vi "FTW-WebServer-Worker.vi"(1 "Endpoint":refnum<class "FTW-Endpoint.lvclass">, 2 "Message Handler":refnum<user-event>) -> ()   [LabVIEW 2015, in "FTW-WebServer.lvclass"]
uses:
  FTW-WebServer.lvclass
  Endpoint/FTW-Endpoint.lvclass
  Message/HttpRequest/FTW-Message-HttpRequest.lvclass
panel:
  out "Messages Handled":u32
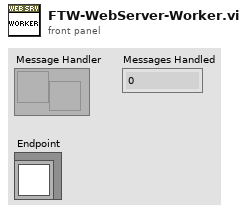
[diagram p1: front panel]
types:
  T1 = typedef "FTW-MessagePayload.ctl" = cluster{"Header":string, "Body":string, "FTW: Sender Identity":string, "FTW: Reply Address":string, "FTW: Reply Error":errorcluster}
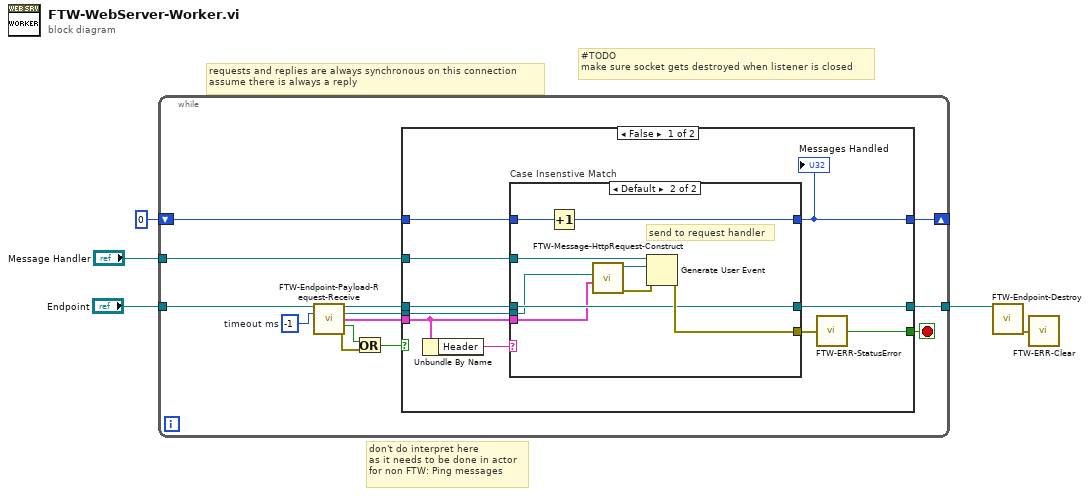
[diagram p0: block diagram]
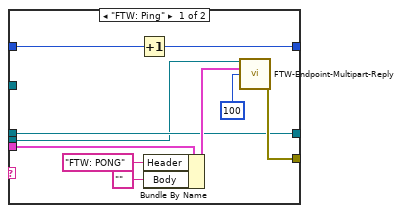
[diagram p2: hidden frame]
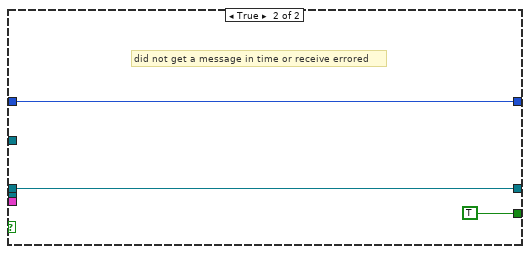
[diagram p3: hidden frame]
diagram:
  # "don't do interpret here\nas it needs to be done in actor\nfor non FTW: Ping messages"
  # "#TODO\nmake sure socket gets destroyed when listener is closed"
  # "requests and replies are always synchronous on this connection\nassume there is always a reply"
  n1 = while {
    tunnel: "Message Handler" -> [w18]
    shift-right: [w11] -> _
    shift-left: u32 0 -> [w12]
    tunnel: "Endpoint" -> [w17]
    tunnel: [w8] -> w3
    stop <- w13 stop-if-true
    w16 = -1  # timeout ms
    n2 = call-dynamic "FTW-Endpoint-Payload-Request-Receive.vi"("FTW Endpoint"=w17, "Timeout"=w16) -> ("FTW Endpoint out"=w10:refnum<class "FTW-Endpoint.lvclass">, "Reply Endpoint"=w14:refnum<class "FTW-Endpoint.lvclass">, "Payload"=w6:T1, "Timed out?"=w7:bool, "error out"=w15:errorcluster)  [unwired: 9 in]
    n3 = Or(x=w7, y=w15) -> (x .or. y?=w9:bool)
    n4 = case shown="False" w9 {
      tunnel: w18 -> [w28 _]
      tunnel: w14 -> [w21 _]
      tunnel: [w24 TRUE] -> w13
      tunnel: w10 -> [w25 w48]
      tunnel: w12 -> [w27 w50]
      tunnel: [w22 w50] -> w11
      tunnel: [w23 w48] -> w8
      tunnel: w6 -> [w20 _]
      frame False {
        n5 = Unbundle By Name(w20) -> ("Header"=w19:string)
        n6 = case "Case Insenstive Match" shown="Default" w19 {
          tunnel: w28 -> [_ w47]
          tunnel: w27 -> [w38 w46]
          tunnel: [w35 w45] -> w22
          tunnel: [w37 w42] -> w26
          tunnel: w25 -> [w31 w41]
          tunnel: w21 -> [w30 w40]
          tunnel: [w31 w41] -> w23
          tunnel: w20 -> [w32 w39]
          frame "FTW: Ping" {
            n7 = Increment(x=w38) -> (x+1=w35:u32)
            n8 = Bundle By Name(cluster=w32, "Header"="FTW: PONG" ("Part"), "Body"="" ("empty string")) -> (w34:T1)
            n9 = call-dynamic "FTW-Endpoint-Multipart-Reply.vi"("FTW Endpoint"=w30, "Message"=w34, "Timeout"=100) -> ("error out"=w37:errorcluster)  [unwired: 10 in, 2 out]
          }
          frame Default {
            # "send to request handler"
            n10 = Increment(x=w46) -> (x+1=w45:u32)
            n11 = call "FTW-Message-HttpRequest-Construct.vi"("Message"=w39, "Frontend Endpoint"=w40) -> ("error out"=w44:errorcluster, "FTW Incoming Request"=w43:refnum<class "FTW-Message-HttpRequest.lvclass">)  [unwired: 8 in]
            n12 = Generate User Event(user event=w47, event data cluster=w43, error in=w44) -> (error out=w42:errorcluster)  [unwired: 1 in, 1 out]
          }
        }
        "Messages Handled" <- w22
        n13 = call "FTW-ERR-StatusError.vi"("error to check"=w26) -> ("Error?"=w24:bool)
      }
      frame True {
        # "did not get a message in time or receive errored"
      }
    }
  }
  n14 = call-dynamic "FTW-Endpoint-Destroy.vi"("FTW Endpoint"=w3) -> ("error out"=w1:errorcluster)  [unwired: 14 in]
  n15 = call "FTW-ERR-Clear.vi"("error to snuff"=w1) -> ()  [unwired: 1 out]
